vi "convert_booleanArray_to_string.vi"(2 "Max Elements Count (All)":i32=-1, 4 "Boolean array in":bool[](array[boolean]), 5 "String to add before (\"\")":string) -> (1 "string out":string)   [LabVIEW 2014, in "rszvl_rsidr_core.lvlib"]
uses:
  rszvl_rsidr_core.lvlib
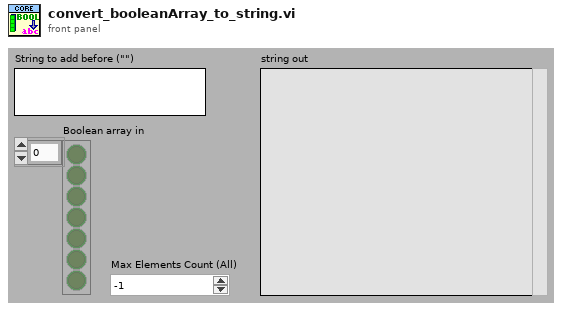
[diagram p1: front panel]
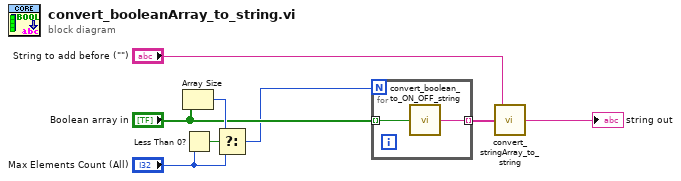
[diagram p0: block diagram]
diagram:
  n1 = Array Size(array="Boolean array in") -> (size(s)=w3:i32)
  n2 = Less Than 0?(x="Max Elements Count (All)") -> (x < 0?=w5:bool)
  n3 = Select(t=w3, s=w5, f="Max Elements Count (All)") -> (s? t:f=w1:i32)
  n4 = for {
    N: w1 -> [_]
    tunnel: "Boolean array in" -> [w10] mode=indexing
    tunnel: [w9] -> w8 mode=indexing
    n5 = call "convert_boolean_to_ON_OFF_string.vi"("boolean value in"=w10) -> ("string value out"=w9:string)  [unwired: 4 in]
  }
  n6 = call "convert_stringArray_to_string.vi"("string array in"=w8, "String to add before (\"\")"="String to add before (\"\")") -> ("string out"=→"string out":string)  [unwired: 3 in]
